vi "X Plus Y.vi"() -> ()   [LabVIEW 2026]
panel:
  out "X+Y":i32=3
  in  "Y":i32=2
  in  "X":i32=1
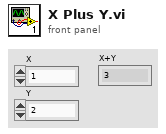
[diagram p1: front panel]
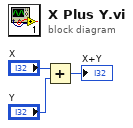
[diagram p0: block diagram]
diagram:
  n1 = Add(x="X", y="Y") -> (x+y=→"X+Y":i32)
